vi "Radar2.vi"() -> ()   [LabVIEW 2017]
panel:
  out "ping":bool
  in  "target coordinates":cluster{"X":i16, "Y":i16}={"X"=-23, "Y"=57}
  in  "stop":bool
  out "2D Picture":picture
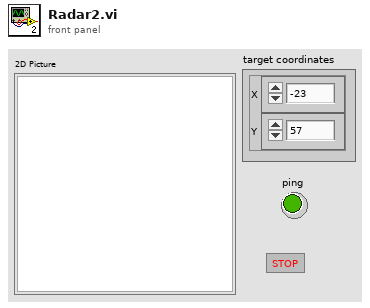
[diagram p1: front panel]
types:
  T1 = cluster{"maximum":dbl, "minimum":dbl, "clip to min":bool, "log?(F)":bool, "grid color":u32, "plot color":u32, "fmt and prec":cluster{"format":enum8{"Decimal", "Scientific", "Engineering", "Binary", "Octal", "Hex"}, "precision":u8}, "visible section":u16}
  T2 = cluster{"Width":u16, "Style":enum32{"Solid", "Dash", "Dot", "DashDot", "DashDotDot"}}
  T3 = typedef "imagedata.ctl" = cluster{"image type":i32, "image depth":i32, "image":u8[], "mask":u8[], "colors":u32[], "Rectangle":cluster{"left":i16, "top":i16, "right":i16, "bottom":i16}}
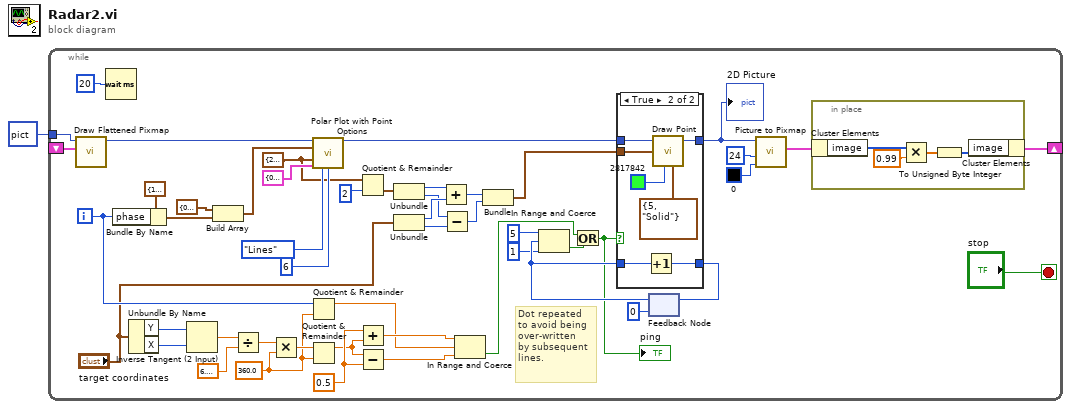
[diagram p0: block diagram]
diagram:
  n1 = while {
    shift-right: [w46] -> _
    shift-left: _ -> [w45]
    tunnel: picture data[5B] ("2D Picture") -> [w44]
    i -> [w25]
    stop <- "stop" stop-if-true
    w32 = 0.5
    w24 = 360.0 ("y")
    w13 = cluster{"width":i16, "height":i16} {"width"=222, "height"=222} ("dimensions (w,h)")
    # "Dot repeated\nto avoid being\nover-written\nby subsequent\nlines."
    n2 = call <vilib>:"Draw Flattened Pixmap.vi"("image data"=w45, "picture"=w44) -> ("new picture"=w51:picture)  [unwired: 7 in]
    n3 = Wait (ms)(milliseconds to wait=u32 20) -> ()  [unwired: 1 out]
    n4 = Bundle By Name(cluster=cluster{"magnitude":dbl, "phase":dbl} {"magnitude"=100.0, "phase"=0.0}, "phase"=w25) -> (w42:cluster{"magnitude":dbl, "phase":dbl})
    n5 = Unbundle By Name("target coordinates") -> ("Y"=w35:i16, "X"=w34:i16)
    n6 = Inverse Tangent (2 Input)(1:w34, 2:w35) -> (0:w29:dbl)
    n7 = Build Array(cluster{"magnitude":dbl, "phase":dbl} {"magnitude"=0.0, "phase"=0.0}, w42) -> (w38:cluster{"magnitude":dbl, "phase":dbl}[])
    n8 = Divide(x=w29, y=6.283185307179586) -> (x/y=w28:dbl)
    n9 = Multiply(x=w28, y=w24) -> (x*y=w27:dbl)
    n10 = Quotient & Remainder(x=w25, y=w24) -> (x-y*floor(x/y)=w23:dbl)  [unwired: 1 out]
    n11 = Quotient & Remainder(x=w27, y=w24) -> (x-y*floor(x/y)=w26:dbl)  [unwired: 1 out]
    n12 = call <vilib>:"Polar Plot with Point Options.vi"("picture"=w51, "data array [mag, phase (deg)]"=w38, "dimensions (w,h)"=w13, "polar attributes"=T1 {"maximum"=0.0, "minimum"=0.0, "clip to min"=FALSE, "log?(F)"=FALSE, "grid color"=6710886, "plot color"=2465536, "fmt and prec"={"format"=enum."Decimal", "precision"=0}, "visible section"=8}, "Lines/Points"=enum16{"Lines", "Points"}."Lines", "Size"=u16 6) -> ("new picture"=w50:picture)  [unwired: 9 in]
    n13 = Quotient & Remainder(x=w13, y=i16 2) -> (floor(x/y)=w19:cluster{"width":i16, "height":i16})  [unwired: 1 out]
    n14 = Add(x=w32, y=w26) -> (x+y=w31:dbl)
    n15 = Subtract(x=w26, y=w32) -> (x-y=w30:dbl)
    n16 = Unbundle(w19) -> ("width"=w18:i16, "height"=w16:i16)
    n17 = Unbundle("target coordinates") -> ("X"=w17:i16, "Y"=w15:i16)
    n18 = Add(x=w18, y=w17) -> (x+y=w14:i16)
    n19 = Subtract(x=w16, y=w15) -> (x-y=w12:i16)
    n20 = In Range and Coerce(upper limit=w31, x=w23, lower limit=w30) -> (In Range?=w6:bool)  [unwired: 1 out]
    n21 = Bundle(w14, w12) -> (w11:cluster{i16, i16})  [unwired: 1 in]
    n22 = feedback #1(u8 0) -> (w5:u8)
    n23 = In Range and Coerce(upper limit=u8 5 ("y"), x=w5, lower limit=u8 1) -> (In Range?=w7:bool)  [unwired: 1 out]
    n24 = Or(x=w6, y=w7) -> (x .or. y?=w2:bool)
    "ping" <- w2
    n25 = case shown="True" w2 {
      tunnel: w50 -> [w52 w59]
      tunnel: [w52 w58] -> w36
      tunnel: w11 -> [_ w57]
      tunnel: [_ w54] -> w9
      tunnel: w5 -> [_ w53]
      frame False {
      }
      frame True {
        n26 = Increment(x=w53) -> (x+1=w54:u8)
        n27 = call <vilib>:"Draw Point.vi"("picture"=w59, "point(x,y)"=w57, "color(black)"=u32 2817842 ("plot color"), "pen"=T2 {"Width"=5, "Style"=enum."Solid"}) -> ("new picture"=w58:picture)  [unwired: 5 in]
      }
    }
    "2D Picture" <- w36
    n28 = feedback-in #1(w9) -> ()
    n29 = call <vilib>:"Picture to Pixmap.vi"("Background Color"=u32 0, "depth"=24, "picture"=w36) -> ("image data"=w47:T3)  [unwired: 7 in, 1 out]
    n30 = in-place {
      n31 = in-place-cluster #2(w47) -> ("image"=w63:u8[])
      n32 = Multiply(x=w63, y=0.99) -> (x*y=w61:dbl[])
      n33 = To Unsigned Byte Integer(number=w61) -> (unsigned 8bit integer=w60:u8[])
      n34 = in-place-cluster #2("image"=w60) -> (w46:T3)
    }
  }
